vi "sonar_output.vi"(7 "stop":bool, 8 "error in":errorcluster, 10 "VCC (default 5)":dbl=5.0, 11 "physical channels":tag) -> (0 "error out":errorcluster, 2 "Output":dbl)   [LabVIEW 2011]
uses:
  <instrlib>/MaxSonar EZ1/driver for Analog/MaxSonar EZ1 Analog (PC).lvlib
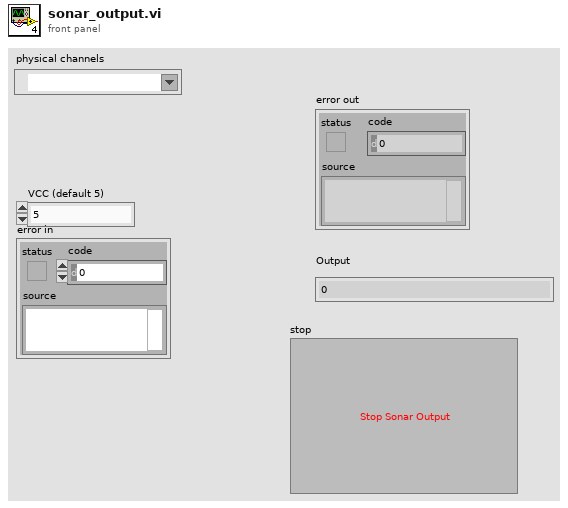
[diagram p1: front panel]
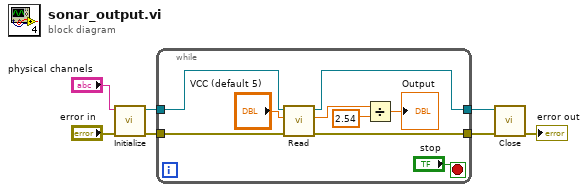
[diagram p0: block diagram]
diagram:
  n1 = call <instrlib>:"Initialize.vi"("error in (no error)"="error in", "physical channels"="physical channels") -> ("error out"=w6:errorcluster, "DAQmx Task Out"=w7:refnum<k21>)  [unwired: 8 in]
  n2 = while {
    tunnel: w7 -> [w16]
    tunnel: w6 -> [w15]
    tunnel: [w14] -> w5
    tunnel: [w13] -> w4
    stop <- "stop" stop-if-true
    n3 = call <instrlib>:"Read.vi"("error in (no error)"=w15, "VCC"="VCC (default 5)", "DAQmx Task Name"=w16) -> ("error out"=w13:errorcluster, "Distance (inch)"=w10:dbl, "DAQmx Task Name Out"=w14:refnum<k21>)  [unwired: 6 in]
    n4 = Divide(x=w10, y=2.54) -> (x/y=→"Output":dbl)
  }
  n5 = call <instrlib>:"Close.vi"("error in (no error)"=w4, "Analog Channel In"=w5) -> ("error out"=→"error out":errorcluster)  [unwired: 9 in]
